vi "get internal stream size.vi"(8 "error in":errorcluster, 11 "connection in":refnum<class "connection.lvclass">) -> (0 "error out":errorcluster, 3 "size":u64)   [LabVIEW 2016, in "connection.lvclass"]
uses:
  connection.lvclass
  connection.lvclass/connection.ctl
  dllwrapper/library path.vi
  dllwrapper/async tls dl.lvlib
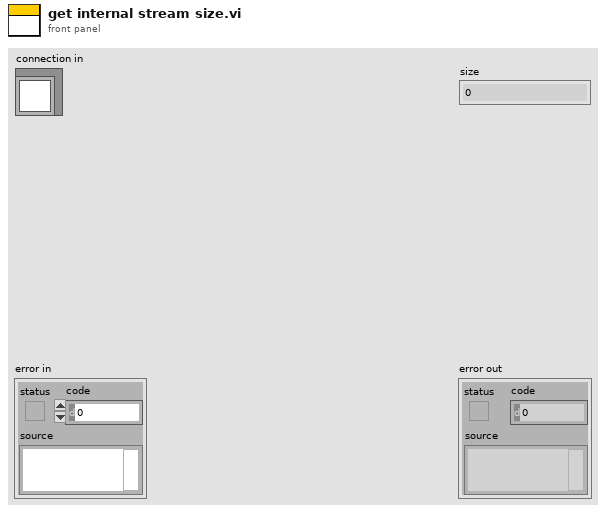
[diagram p1: front panel]
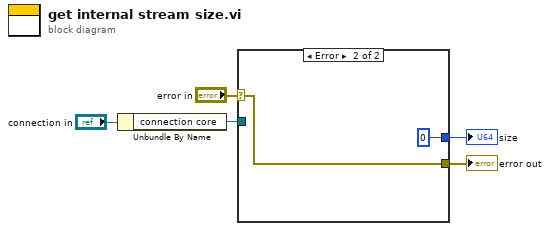
[diagram p0: block diagram]
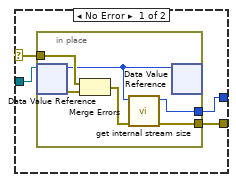
[diagram p2: hidden frame]
diagram:
  n1 = Unbundle By Name("connection in") -> ("connection core"=w4:refnum<data-value>)
  n2 = case shown="Error" "error in" {
    selector: "error in" -> [w8 w17]
    tunnel: w4 -> [w9 _]
    tunnel: [w7 w17] -> w2
    tunnel: [w6 u64 0 ("size")] -> w1
    frame No Error {
      n3 = in-place {
        in-place-border: w8 -> [w15]
        in-place-border: [w12] -> w7
        in-place-border: [w10] -> w6
        n4 = in-place-dvr #1(w9) -> (w11:u64, w14:errorcluster)
        n5 = Merge Errors(w15, w14) -> (w13:errorcluster)
        n6 = call "get internal stream size.vi"("error im"=w13, "socket"=w11) -> ("error out"=w12:errorcluster, "size"=w10:u64)  [unwired: 8 in]
        n7 = in-place-dvr #1(w11) -> ()  [unwired: 2 out]
      }
    }
    frame Error {
    }
  }
  "error out" <- w2
  "size" <- w1
